vi "alignBottom.vi"(8 "error in (no error)":errorcluster, 11 "refs":refnum<vi>[](array[refnum])) -> (0 "error out":errorcluster, 3 "refs(dup)":refnum<vi>[](array[refnum]))   [LabVIEW 2023, in "TLC_Geometry.lvlib"]
doc: "Aligns all controls to the topmost position among the input controls.\nThe topmost coordinate is computed and applied to all controls."
uses:
  TLC_Geometry.lvlib
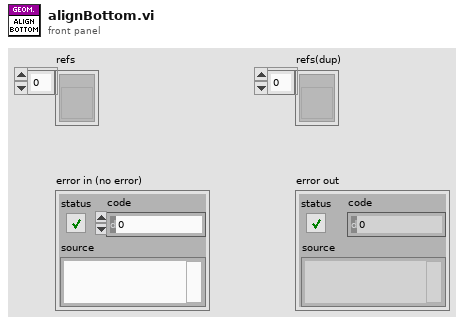
[diagram p1: front panel]
types:
  T1 = cluster{"left":i32, "top":i32, "right":i32, "bottom":i32}
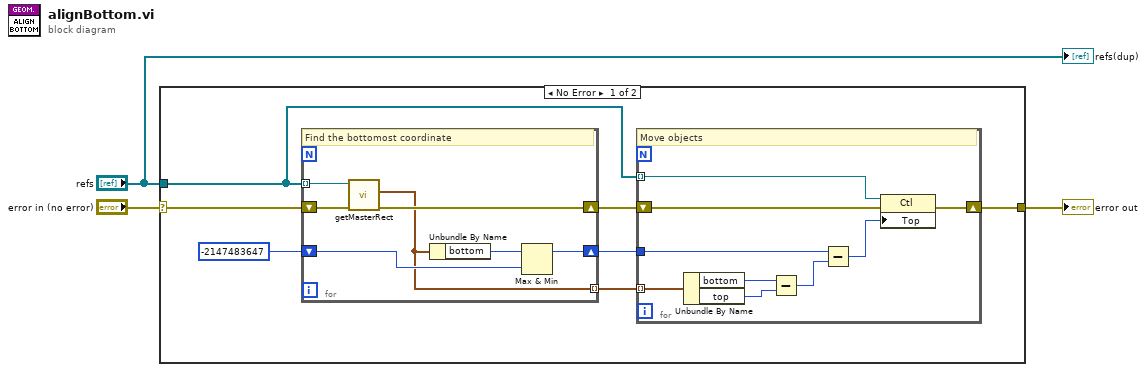
[diagram p0: block diagram]
diagram:
  n1 = case shown="No Error" "error in (no error)" {
    selector: "error in (no error)" -> [w10 w27]
    tunnel: [w7 w27] -> w2
    tunnel: "refs" -> [w8 _]
    frame No Error {
      n2 = for {
        tunnel: w8 -> [w26] mode=indexing
        shift-right: [w24] -> w6
        shift-left: w10 -> [w25]
        shift-right: [w21] -> w5
        shift-left: -2147483647 -> [w22]
        tunnel: [w20] -> w4 mode=indexing
        # "Find the bottomost coordinate"
        n3 = call "getMasterRect.vi"("error in (no error)"=w25, "ref"=w26) -> ("error out"=w24:errorcluster, "rect"=w20:T1)  [unwired: 7 in, 1 out]
        n4 = Unbundle By Name(w20) -> ("bottom"=w23:i32)
        n5 = Max & Min(x=w23, y=w22) -> (max(x,y)=w21:i32)  [unwired: 1 out]
      }
      n6 = for {
        tunnel: w8 -> [w19] mode=indexing
        shift-right: [w17] -> w7
        shift-left: w6 -> [w18]
        tunnel: w5 -> [w13]
        tunnel: w4 -> [w16] mode=indexing
        # "Move objects"
        n7 = Unbundle By Name(w16) -> ("bottom"=w15:i32, "top"=w14:i32)
        n8 = Subtract(x=w15, y=w14) -> (x-y=w12:i32)
        n9 = Subtract(x=w13, y=w12) -> (x-y=w11:i32)
        n10 = property class="Ctl"(reference=w19, error in=w18, "Top"=w11) -> (error out=w17:errorcluster)  [unwired: 1 out]
      }
    }
    frame Error {
    }
  }
  "error out" <- w2
  "refs(dup)" <- "refs"
